vi "ElevatorSafetyInterlocks.vi"(8 "Feed Forward Contribution":dbl, 9 "Elevator State In":string, 10 "Elevator Power In":dbl) -> (1 "Elevator State Out":string, 2 "Elevator Power Out":dbl)   [LabVIEW 2018]
uses:
  Inputs_DriverStation.vi
  SensorReadings.vi
  RobotStates.vi
panel:
  in  "Ignore Stall Safety (in)":dbl=85.0
  in  "Maximum (Climbing) Elevator Height (in)":dbl=65.0
  in  "Encoder Check Velocity (in/s)":dbl=0.1 format="%#_13g"
  in  "Maximum (Normal) Elevator Height (in)":dbl=92.0
  in  "Encoder Check Delay (ms)":u32=3000
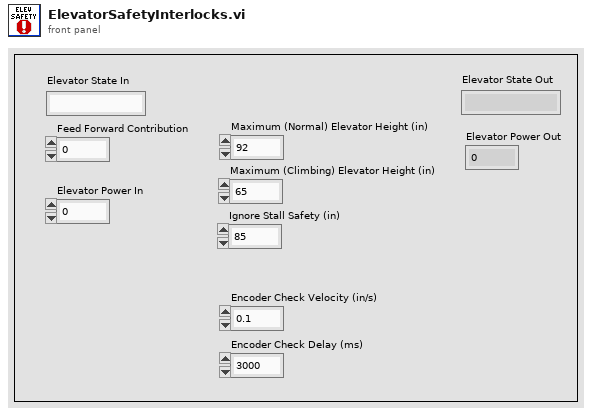
[diagram p1: front panel]
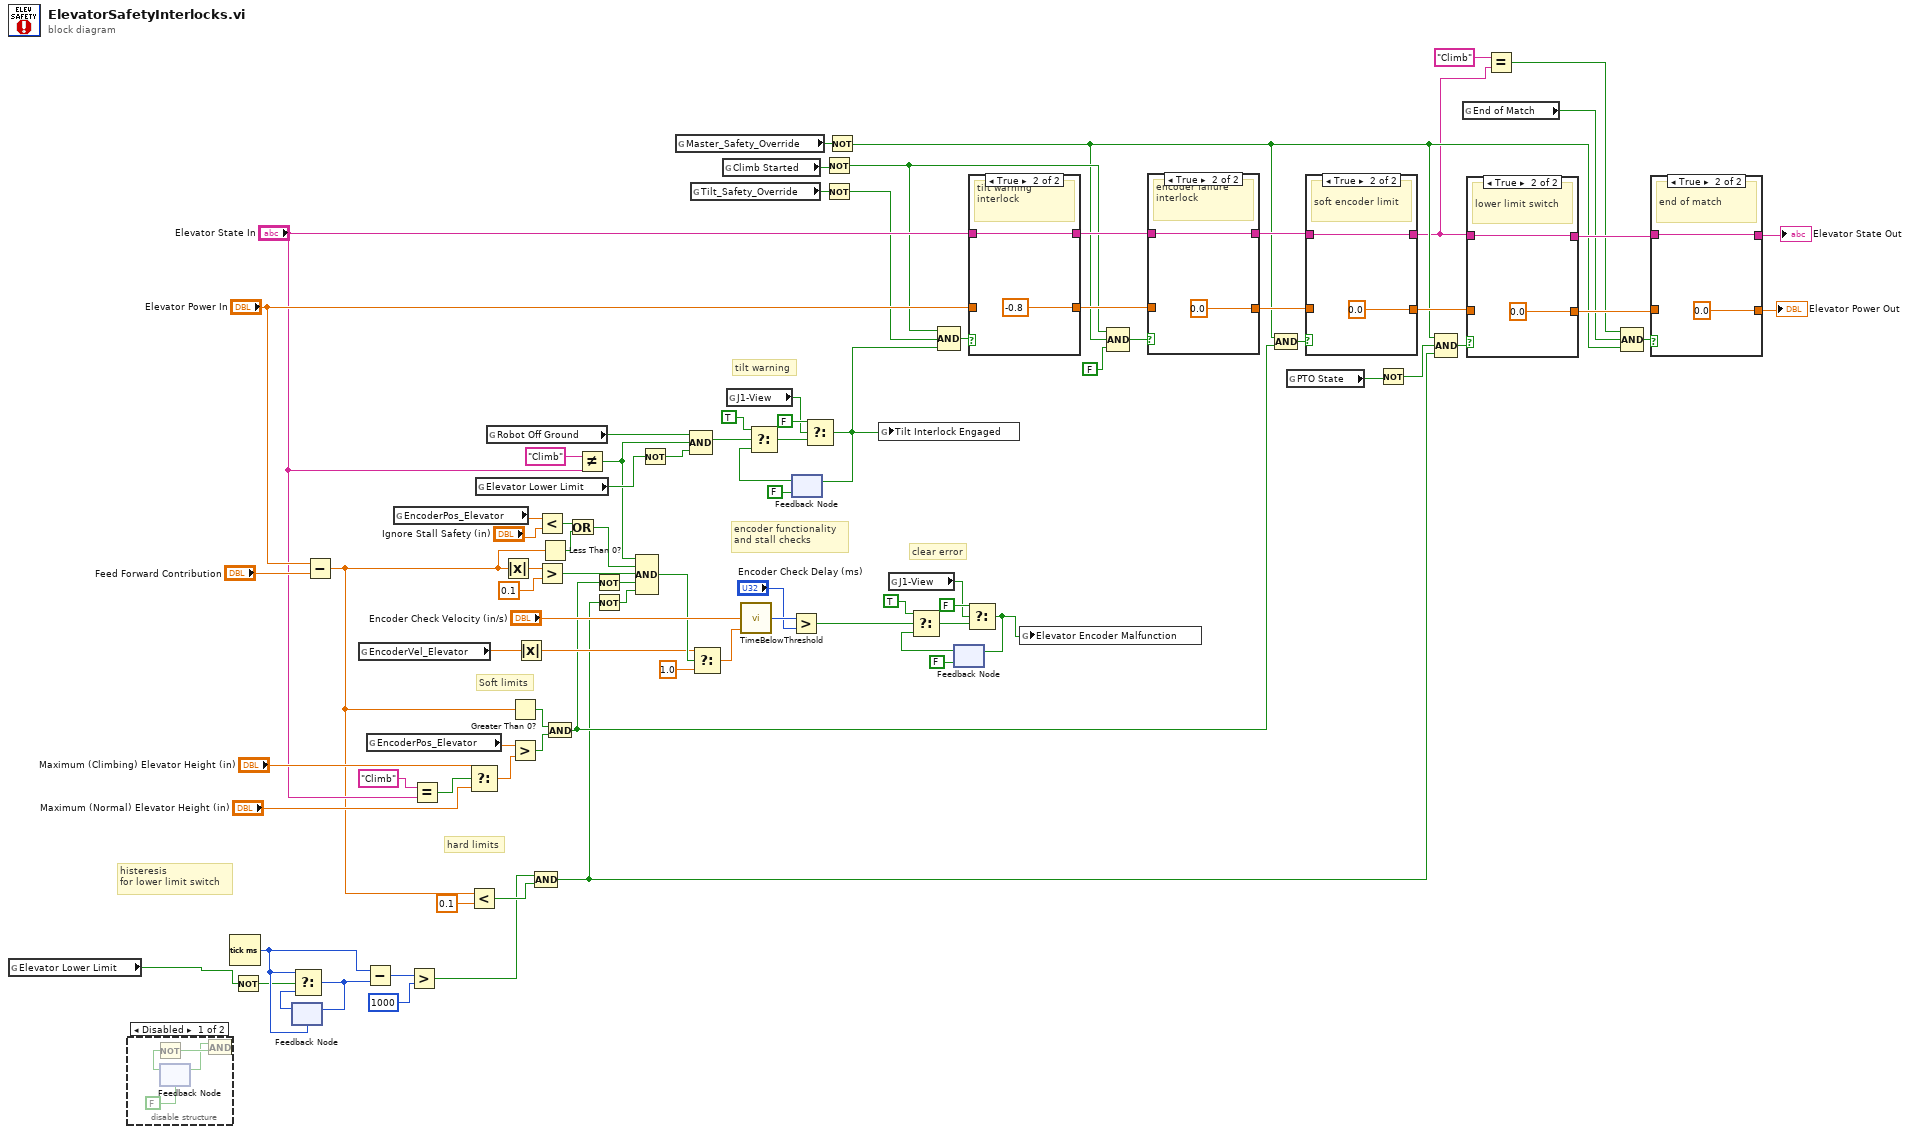
[diagram p0: block diagram]
diagram:
  # "histeresis\nfor lower limit switch"
  # "clear error"
  # "tilt warning"
  # "hard limits"
  # "Soft limits"
  # "encoder functionality\nand stall checks"
  n1 = global read "SensorReadings.vi" "Elevator Lower Limit"() -> (w1:bool)
  n2 = disable-structure shown="Disabled" {
    frame Disabled {
      n3 = feedback #1(FALSE ("Elevator Lower Limit")) -> (w94:bool)
      n4 = Not(x=w94) -> (.not. x?=w93:bool)
      n5 = feedback-in #1() -> (w91:bool)
      n6 = And(x=w91, y=w93) -> ()  [unwired: 1 out]
    }
    frame Enabled {
    }
  }
  n7 = Tick Count (ms)() -> (millisecond timer value=w6:u32)
  n8 = Not(x=w1) -> (.not. x?=w2:bool)
  n9 = feedback #2(w6) -> (w8:u32)
  n10 = Select(t=w6, s=w2, f=w8) -> (s? t:f=w7:u32)
  n11 = feedback-in #2(w7) -> ()
  n12 = Subtract(x="Elevator Power In", y="Feed Forward Contribution") -> (x-y=w23:dbl)
  n13 = global read "SensorReadings.vi" "EncoderVel_Elevator"() -> (w89:dbl)
  n14 = Subtract(x=w6, y=w7) -> (x-y=w5:u32)
  n15 = global read "SensorReadings.vi" "EncoderPos_Elevator"() -> (w83:dbl)
  n16 = global read "SensorReadings.vi" "EncoderPos_Elevator"() -> (w28:dbl)
  n17 = Greater?(x=w5, y=u32 1000) -> (0:w3:bool)
  n18 = Equal?(x="Climb", y="Elevator State In") -> (x = y?=w49:bool)
  n19 = Select(t="Maximum (Climbing) Elevator Height (in)", s=w49, f="Maximum (Normal) Elevator Height (in)") -> (s? t:f=w55:dbl)
  n20 = Less?(x=w23, y=0.1) -> (x < y?=w65:bool)
  n21 = global read "SensorReadings.vi" "Elevator Lower Limit"() -> (w51:bool)
  n22 = global read "SensorReadings.vi" "Robot Off Ground"() -> (w52:bool)
  n23 = Absolute Value(x=w23) -> (abs(x)=w43:dbl)
  n24 = Greater Than 0?(x=w23) -> (x > 0?=w82:bool)
  n25 = Greater?(x=w83, y=w55) -> (0:w81:bool)
  n26 = Absolute Value(x=w89) -> (abs(x)=w35:dbl)
  n27 = Compound Arithmetic op=AND(w3, w65) -> (w29:bool)
  n28 = Less?(x=w28, y="Ignore Stall Safety (in)") -> (x < y?=w26:bool)
  n29 = Greater?(x=w43, y=0.1) -> (0:w39:bool)
  n30 = Less Than 0?(x=w23) -> (x < 0?=w24:bool)
  n31 = And(x=w82, y=w81) -> (x .and. y?=w31:bool)
  n32 = Or(x=w26, y=w24) -> (x .or. y?=w25:bool)
  n33 = Not Equal?(x="Climb", y="Elevator State In") -> (x != y?=w11:bool)
  n34 = Not(x=w31) -> (.not. x?=w38:bool)
  n35 = Not(x=w29) -> (.not. x?=w32:bool)
  n36 = Compound Arithmetic op=AND(w11, w25, w39, w38, w32) -> (w36:bool)
  n37 = Not(x=w51) -> (.not. x?=w46:bool)
  n38 = global read "Inputs_DriverStation.vi" "Master_Safety_Override"() -> (w90:bool)
  n39 = Compound Arithmetic op=AND(w52, w11, w46) -> (w69:bool)
  n40 = global read "Inputs_DriverStation.vi" "Tilt_Safety_Override"() -> (w10:bool)
  n41 = Select(t=w35, s=w36, f=1.0) -> (s? t:f=w37:dbl)
  n42 = global read "RobotStates.vi" "Climb Started"() -> (w54:bool)
  n43 = global read "Inputs_DriverStation.vi" "J1-View"() -> (w73:bool)
  n44 = call "TimeBelowThreshold.vi"("Current Value"=w37, "Threshold"="Encoder Check Velocity (in/s)") -> ("Time Below"=w86:u32)  [unwired: 3 in]
  n45 = Greater?(x=w86, y="Encoder Check Delay (ms)") -> (0:w41:bool)
  n46 = feedback #3(FALSE) -> (w77:bool)
  n47 = Select(t=TRUE, s=w69, f=w77) -> (s? t:f=w75:bool)
  n48 = Select(t=FALSE, s=w73, f=w75) -> (s? t:f=w45:bool)
  n49 = feedback-in #3(w45) -> ()
  n50 = Not(x=w54) -> (.not. x?=w47:bool)
  n51 = Not(x=w10) -> (.not. x?=w9:bool)
  n52 = Not(x=w90) -> (.not. x?=w16:bool)
  n53 = global write "RobotStates.vi" "Tilt Interlock Engaged"(w45) -> ()
  n54 = global read "Inputs_DriverStation.vi" "J1-View"() -> (w58:bool)
  n55 = Compound Arithmetic op=AND(w47, w9, w45) -> (w64:bool)
  n56 = feedback #4(FALSE) -> (w62:bool)
  n57 = Select(t=TRUE, s=w41, f=w62) -> (s? t:f=w60:bool)
  n58 = Select(t=FALSE, s=w58, f=w60) -> (s? t:f=w33:bool)
  n59 = feedback-in #4(w33) -> ()
  n60 = case shown="True" w64 {
    tunnel: [w95 -0.8 ("Elevator Power In")] -> w70
    tunnel: "Elevator State In" -> [w96 w97]
    tunnel: [w96 w97] -> w72
    tunnel: "Elevator Power In" -> [w95 _]
    frame False {
      # "tilt okay"
    }
    frame True {
      # "tilt warning interlock"
    }
  }
  n61 = global write "SensorReadings.vi" "Elevator Encoder Malfunction"(w33) -> ()
  n62 = Compound Arithmetic op=AND(w47, w16, FALSE) -> (w44:bool)
  n63 = case shown="True" w44 {
    tunnel: [w99 0.0 ("Elevator Power In")] -> w84
    tunnel: w70 -> [w99 _]
    tunnel: [w100 w102] -> w85
    tunnel: w72 -> [w100 w102]
    frame False {
      # "okay encoder"
    }
    frame True {
      # "encoder failure interlock"
    }
  }
  n64 = Compound Arithmetic op=AND(w16, w31) -> (w67:bool)
  n65 = global read "RobotStates.vi" "PTO State"() -> (w53:bool)
  n66 = case shown="True" w67 {
    tunnel: [w103 0.0 ("Elevator Power In")] -> w80
    tunnel: w84 -> [w103 _]
    tunnel: [w104 w106] -> w14
    tunnel: w85 -> [w104 w106]
    frame False {
      # "okay height"
    }
    frame True {
      # "soft encoder limit"
    }
  }
  n67 = Not(x=w53) -> (.not. x?=w30:bool)
  n68 = Compound Arithmetic op=AND(w16, w30, w29) -> (w66:bool)
  n69 = global read "RobotStates.vi" "End of Match"() -> (w13:bool)
  n70 = case shown="True" w66 {
    tunnel: [w107 0.0 ("Elevator Power In")] -> w20
    tunnel: w80 -> [w107 _]
    tunnel: [w108 w110] -> w21
    tunnel: w14 -> [w108 w110]
    frame False {
      # "okay lower limit switch"
    }
    frame True {
      # "lower limit switch"
    }
  }
  n71 = Equal?(x="Climb", y=w14) -> (x = y?=w12:bool)
  n72 = Compound Arithmetic op=AND(w12, w13, w16) -> (w17:bool)
  n73 = case shown="True" w17 {
    tunnel: [w111 0.0 ("Elevator Power In")] -> w18
    tunnel: w20 -> [w111 _]
    tunnel: [w112 w114] -> w19
    tunnel: w21 -> [w112 w114]
    frame False {
      # "not end of match"
    }
    frame True {
      # "end of match"
    }
  }
  "Elevator Power Out" <- w18
  "Elevator State Out" <- w19
